vi "Actor - SEND - Triggered Event.vi"(7 "Actor Selector":T1, 8 "error in (no error)":errorcluster, 9 "Data":string="Hi!!!", 10 "Events":T2=enum."START Ev") -> (0 "error out":errorcluster)   [LabVIEW 2023, in "Controller.lvlib" / "Controller.lvclass"]
uses:
  Controller.lvclass
  GUI/Usr Ev/GUI - Ctrl - Enum - Events.ctl
  Controller - Ctrl - Actor - Selector.ctl
  Message_Distributor/Message_Distributor_Class.lvclass
  C:/Users/rodri/LabVIEW_Labs/LabVIEW_GitHub/LV_AF_Project/AF_Architecture/Abstraction_Interface_Class/Abstraction_Interface_Class.lvclass
  GUI/GUI_Class.lvclass
  Console/Console_Class.lvclass
  SW_Interface/SW_Interface_Class.lvclass
  Controller - Ctrl - FGV - Action.ctl
  Logging/Logging_Class.lvclass
  Error_Engine/Error_Emgime_Class.lvclass
  Embedded_DB/Embedded_DB_Class.lvclass
  Message_Distributor/Distributor_Class Messages/Distributor - SEND - Triggered Event Msg/Distributor - SEND - Triggered Event Msg.lvclass/Distributor - SEND - Triggered Event Msg.ctl
  <vilib>/ActorFramework/Message Enqueuer/Message Enqueuer.lvclass/Message Enqueuer.ctl
  <vilib>/ActorFramework/Message Enqueuer/Enqueue.vi
  Message_Distributor/Distributor_Class Messages/Distributor - SEND - Triggered Event Msg/Distributor - SEND - Triggered Event Msg.lvclass
  C:/Program Files/National Instruments/LabVIEW 2023/vi.lib/ActorFramework/Message/Message.lvclass
  <vilib>/ActorFramework/Message Priority Queue/Priority Enqueue.vi
  Abstraction_Interface_Class/Abstraction_Interface_Class.lvclass
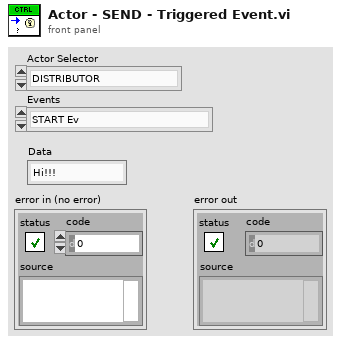
[diagram p1: front panel]
types:
  T1 = typedef "Controller.lvlib/Controller.lvclass/Controller - Ctrl - Actor - Selector.ctl" = enum16{"DISTRIBUTOR", "GUI", "CONSOLE", "SW_INTERFACE", "LOGGING", "ERROR_ENGINE", "EMBEDDED_DB"}
  T2 = typedef "GUI_Actor.lvlib/GUI_Class.lvclass/GUI - Ctrl - Enum - Events.ctl" = enum16{"SEND MESSAGE Ev", "STOP_ACTOR Ev", "INIT_ACTOR Ev", "START Ev", "STOP Ev", "GET Ev", "SET Ev", "ERROR_HANDLER Ev", "RESET Ev", "T2 Ev", "T3 Ev", "T4 Ev"}
  T3 = typedef "Controller.lvlib/Controller.lvclass/Controller - Ctrl - FGV - Action.ctl" = enum16{"Int", "Get"}
  T4 = map{string, refnum<class "Abstraction_Interface_Class.lvclass">}
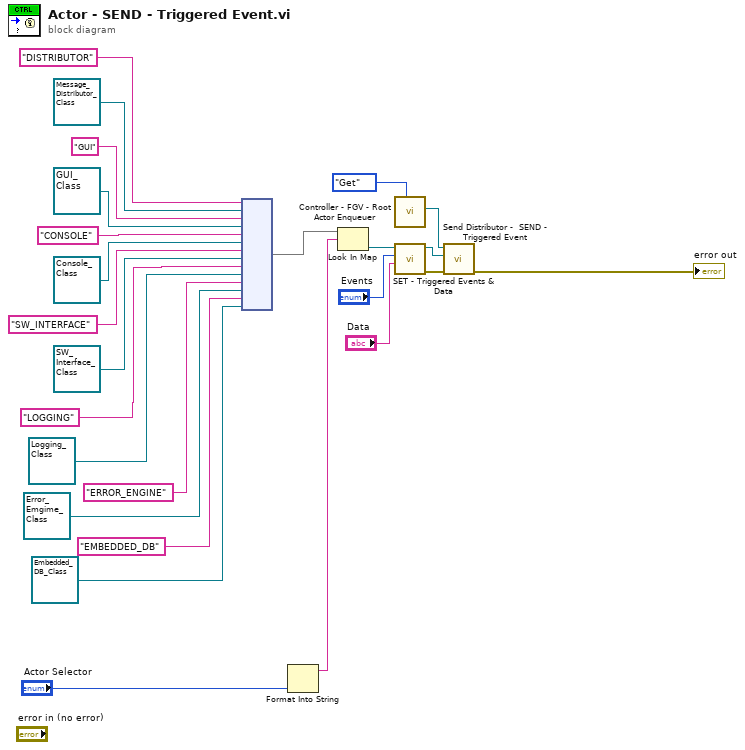
[diagram p0: block diagram]
diagram:
  n1 = node("DISTRIBUTOR" ("key"), refnum<class "Message_Distributor_Class.lvclass"> refnum ("Actor_Parent.lvlib:Parent_Class.lvclass"), "GUI" ("key"), refnum<class "GUI_Class.lvclass"> refnum ("Actor_Child_1.lvlib:Child_1_Class.lvclass"), "CONSOLE" ("key"), refnum<class "Console_Class.lvclass"> refnum ("Actor_Child_2.lvlib:Child_2_Class.lvclass"), "SW_INTERFACE" ("key"), refnum<class "SW_Interface_Class.lvclass"> refnum ("Actor_Child_3.lvlib:Child_3_Class.lvclass"), "LOGGING" ("key"), refnum<class "Logging_Class.lvclass"> refnum ("Logging.lvlib:Logging_Class.lvclass"), "ERROR_ENGINE" ("Actor_Name IN"), refnum<class "Error_Emgime_Class.lvclass"> refnum ("Error_Engine_Actor.lvlib:Error_Emgime_Class.lvclass"), "EMBEDDED_DB" ("Actor_Name IN"), refnum<class "Embedded_DB_Class.lvclass"> refnum ("Embedded_DB_Actor.lvlib:Embedded_DB_Class.lvclass")) -> (w18:T4)
  n2 = Format Into String("Actor Selector") -> (resulting string=w16:string)  [unwired: 3 in, 1 out]
  n3 = Look In Map(map=w18, key=w16) -> (value=w14:refnum<class "Abstraction_Interface_Class.lvclass">)  [unwired: 1 in, 1 out]
  n4 = call "Controller - FGV - Root Actor Enqueuer.vi"("Action"=Controller_-_Ctrl_-_FGV_-_Action."Get") -> ("Root Enqueuer"=w15:refnum<class "Message Enqueuer.lvclass">)  [unwired: 9 in, 1 out]
  n5 = call-dynamic "SET - Triggered Events & Data.vi"("Data"="Data", "Events"="Events", "Interface_Class in"=w14) -> ("error out"=w11:errorcluster, "Interface_Class out"=w10:refnum<class "Abstraction_Interface_Class.lvclass">)  [unwired: 7 in]
  n6 = call "Send Distributor -  SEND - Triggered Event.vi"("error in (no error)"=w11, "Actor_Interface.lvlib:Interface_Class.lvclass"=w10, "Message Enqueuer"=w15) -> ("error out"=→"error out":errorcluster)  [unwired: 7 in, 1 out]
